vi "Warning Dialog Main.vi"(8 "error in (no error)":errorcluster, 11 "Message in":string) -> (0 "error out":errorcluster)   [LabVIEW 2015, in "Warning Dialog.lvclass"]
doc: "<b> </b> <b> </b>\n©2016 Q Software Innovations, LLC (QSI)\nwritten by Quentin Alldredge\nproduced in LabVIEW 2015\n\nsupport@qsoftwareinnovations.com\nwww.qsoftwareinnovations.com\n\nAll rights reserved.\n\nRedistribution and use in source and binary forms, with or without modification, are permitted provided that the following conditions are met:\n\n * Redistributions of source code must retain the above copyright notice, this list of conditions and the following disclaimer.\n * Redistributions in binary form must reproduce the above copyright notice, this list of conditions and the following disclaimer in the documentation and/or other materials provided with the distribution.\n * Neither the name of Q Software Innovations, LLC. nor the names of its contributors may be used to endorse or promote products derived from this software without specific prior written permission.\n\nTHIS SOFTWARE IS PROVIDED BY THE COPYRIGHT HOLDERS AND CONTRIBUTORS \"AS IS\" AND ANY EXPRESS OR IMPLIED WARRANTIES, INCLUDING, BUT NOT LIMITED TO, THE IMPLIED WARRANTIES OF MERCHANTABILITY AND FITNESS FOR A PARTICULAR PURPOSE ARE DISCLAIMED. IN NO EVENT SHALL THE COPYRIGHT OWNER OR CONTRIBUTORS BE LIABLE FOR ANY DIRECT, INDIRECT, INCIDENTAL, SPECIAL, EXEMPLARY, OR CONSEQUENTIAL DAMAGES (INCLUDING, BUT NOT LIMITED TO, PROCUREMENT OF SUBSTITUTE GOODS OR SERVICES; LOSS OF USE, DATA, OR PROFITS; OR BUSINESS INTERRUPTION) HOWEVER CAUSED AND ON ANY THEORY OF LIABILITY, WHETHER IN CONTRACT, STRICT LIABILITY, OR TORT (INCLUDING NEGLIGENCE OR OTHERWISE) ARISING IN ANY WAY OUT OF THE USE OF THIS SOFTWARE, EVEN IF ADVISED OF THE POSSIBILITY OF SUCH DAMAGE."
uses:
  Warning Dialog.lvclass
  Dialog/Dialog.lvclass
panel:
  in  "OK":bool
  out "Message":string
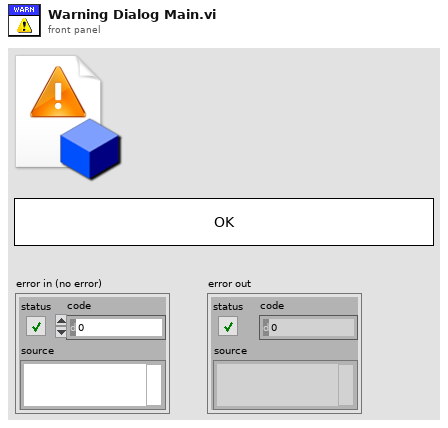
[diagram p1: front panel]
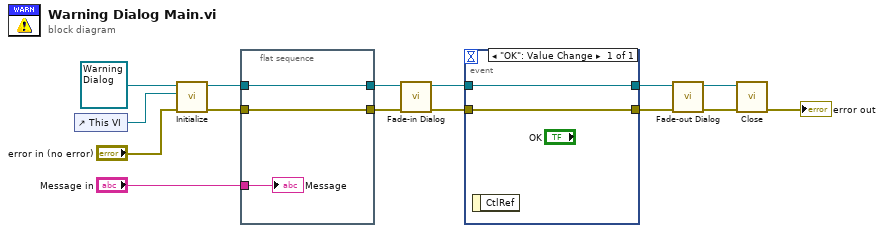
[diagram p0: block diagram]
diagram:
  n1 = control-ref of="This VI"() -> (w14:refnum<vi>)
  n2 = call-dynamic "Initialize.vi"("error in (no error)"="error in (no error)", "VI Refnum"=w14, "Warning Dialog in"=refnum<class "Warning Dialog.lvclass"> refnum ("Warning")) -> ("error out"=w9:errorcluster, "Warning Dialog out"=w11:refnum<class "Warning Dialog.lvclass">)  [unwired: 7 in]
  n3 = flat-sequence {
    tunnel: "Message in" -> [w18]
    tunnel: [w17] -> w12
    tunnel: w11 -> [w17]
    tunnel: [w16] -> w10
    tunnel: w9 -> [w16]
    frame #0 {
      "Message" <- w18
    }
  }
  n4 = call "Fade-in Dialog.vi"("error in (no error)"=w10, "Dialog in"=w12) -> ("error out"=w8:errorcluster, "Dialog out"=w7:refnum<class "Warning Dialog.lvclass">)  [unwired: 8 in]
  n5 = event shown="[0] \"OK\": Value Change" {
    selector: _ -> [_]
    dyn-events: _ -> [_]
    timeout: _ -> [_]
    tunnel: w8 -> [w19]
    tunnel: w7 -> [w20]
    tunnel: [w20] -> w6
    tunnel: [w19] -> w5
    event "OK": Value Change {
      n6 = event-data() -> ()  [unwired: 1 in, 1 out]
    }
  }
  n7 = call "Fade-out Dialog.vi"("error in (no error)"=w5, "Dialog in"=w6) -> ("error out"=w3:errorcluster, "Dialog out"=w4:refnum<class "Warning Dialog.lvclass">)  [unwired: 8 in]
  n8 = call-dynamic "Close.vi"("error in (no error)"=w3, "Dialog in"=w4) -> ("error out"=→"error out":errorcluster)  [unwired: 9 in]
